vi "Write step demand.vi"(10 "step demand":dbl=5000.0 min=10.0 max=5000.0, 11 "StepperMotor in":refnum<class "StepperMotor.lvclass">) -> (3 "StepperMotor out":refnum<class "StepperMotor.lvclass">)   [LabVIEW 2013, in "StepperMotor.lvclass"]
uses:
  StepperMotor.lvclass
  StepperMotor.lvclass/StepperMotor.ctl
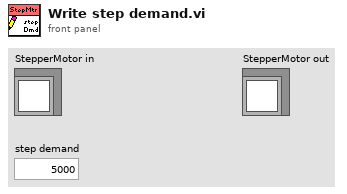
[diagram p1: front panel]
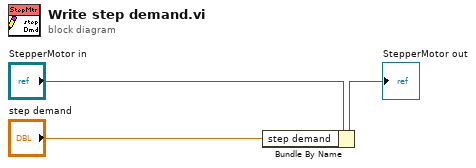
[diagram p0: block diagram]
diagram:
  n1 = Bundle By Name(cluster="StepperMotor in", "step demand"="step demand") -> (→"StepperMotor out":refnum<class "StepperMotor.lvclass">)
